vi "check_login.vi"(8 "error in (no error)":errorcluster, 9 "password":string, 10 "username":string, 11 "DB Session ID":i32) -> (0 "error out":errorcluster, 3 "DB Session ID out":i32)   [LabVIEW 2022 SP3, in "Database.lvlib"]
uses:
  Database.lvlib
  bin/Database.dll
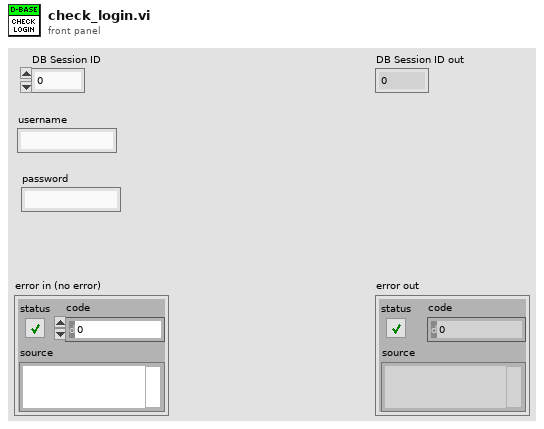
[diagram p1: front panel]
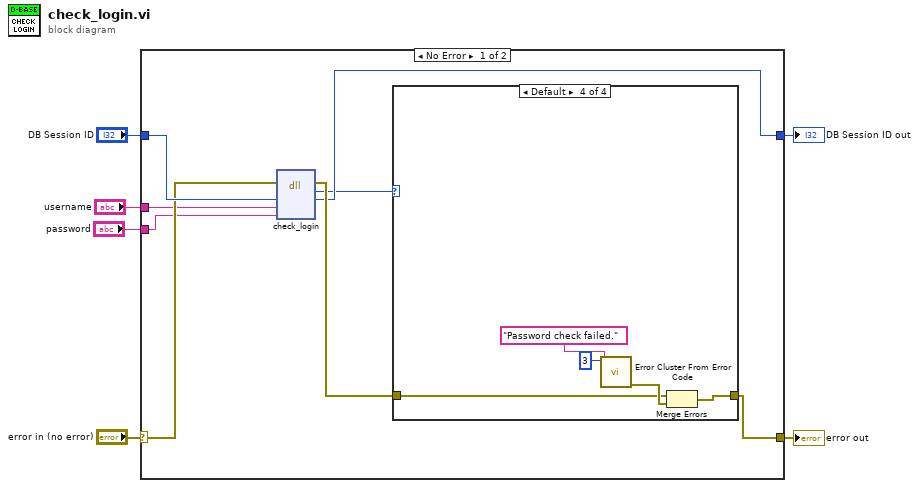
[diagram p0: block diagram]
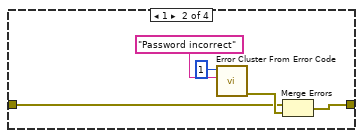
[diagram p3: hidden frame]
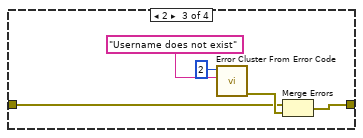
[diagram p4: hidden frame]
diagram:
  n1 = case shown="No Error" "error in (no error)" {
    selector: "error in (no error)" -> [w12 w32]
    tunnel: [w11 w32] -> w4
    tunnel: "DB Session ID" -> [w13 w31]
    tunnel: [w10 w31] -> w3
    tunnel: "username" -> [w9 _]
    tunnel: "password" -> [w8 _]
    frame No Error {
      n2 = dll-call lib="C:/Users/Caleb/Desktop/nebraska-silicon-lab/pixel-gantry-control/Gantry/Shared Components/bin/Database.dll" fn="check_login"(error in=w12, "session_id"=w13, "username"=w9, "password"=w8) -> (error out=w14:errorcluster, "return type"=w7:i32, "session_id"=w10:i32)  [unwired: 4 in, 1 out]
      n3 = case shown="Default" w7 {
        tunnel: w14 -> [w15 w18 w23 w28]
        tunnel: [w15 w17 w22 w27] -> w11
        frame 0 {
          # "Ok"
        }
        frame 1 {
          n4 = call <vilib>:"Error Cluster From Error Code.vi"("error message (\"\")"="Password incorrect" ("error message (\"\")"), "error code (0)"=1) -> ("error out"=w20:errorcluster)  [unwired: 7 in]
          n5 = Merge Errors(w18, w20) -> (w17:errorcluster)
        }
        frame 2 {
          n6 = call <vilib>:"Error Cluster From Error Code.vi"("error message (\"\")"="Username does not exist" ("error message (\"\")"), "error code (0)"=2) -> ("error out"=w25:errorcluster)  [unwired: 7 in]
          n7 = Merge Errors(w23, w25) -> (w22:errorcluster)
        }
        frame Default {
          n8 = call <vilib>:"Error Cluster From Error Code.vi"("error message (\"\")"="Password check failed." ("error message (\"\")"), "error code (0)"=3) -> ("error out"=w30:errorcluster)  [unwired: 7 in]
          n9 = Merge Errors(w28, w30) -> (w27:errorcluster)
        }
      }
    }
    frame Error {
    }
  }
  "error out" <- w4
  "DB Session ID out" <- w3
